vi "GetAppRefInClusterArray.vi"() -> (0 "error out":errorcluster, 1 "Array":cluster{"App Refnum":refnum<vi>}[](array[cluster]))   [LabVIEW 2010]
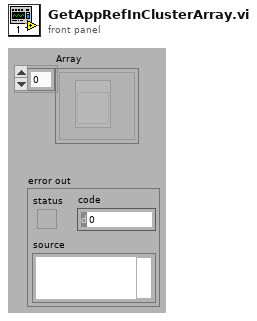
[diagram p1: front panel]
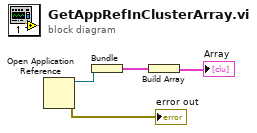
[diagram p0: block diagram]
diagram:
  n1 = Open Application Reference() -> (0:→"error out":errorcluster, 3:w3:refnum<vi>)  [unwired: 1 in, 3 out]
  n2 = Bundle("application reference"=w3) -> (w1:cluster{"application reference":refnum<vi>})  [unwired: 1 in]
  n3 = Build Array(w1) -> (→"Array":cluster{"application reference":refnum<vi>}[])
